vi "test.vi"() -> ()   [LabVIEW 2013]
uses:
  RydbergExpControl/red_mot_controls.ctl
  <vilib>/NI/GXML/GXML.lvlib
panel:
  out "error out":errorcluster
  in  "XML File Path":path
  in  "Inputs":T1 {"Waveform Parameters"."Degree" min=1}
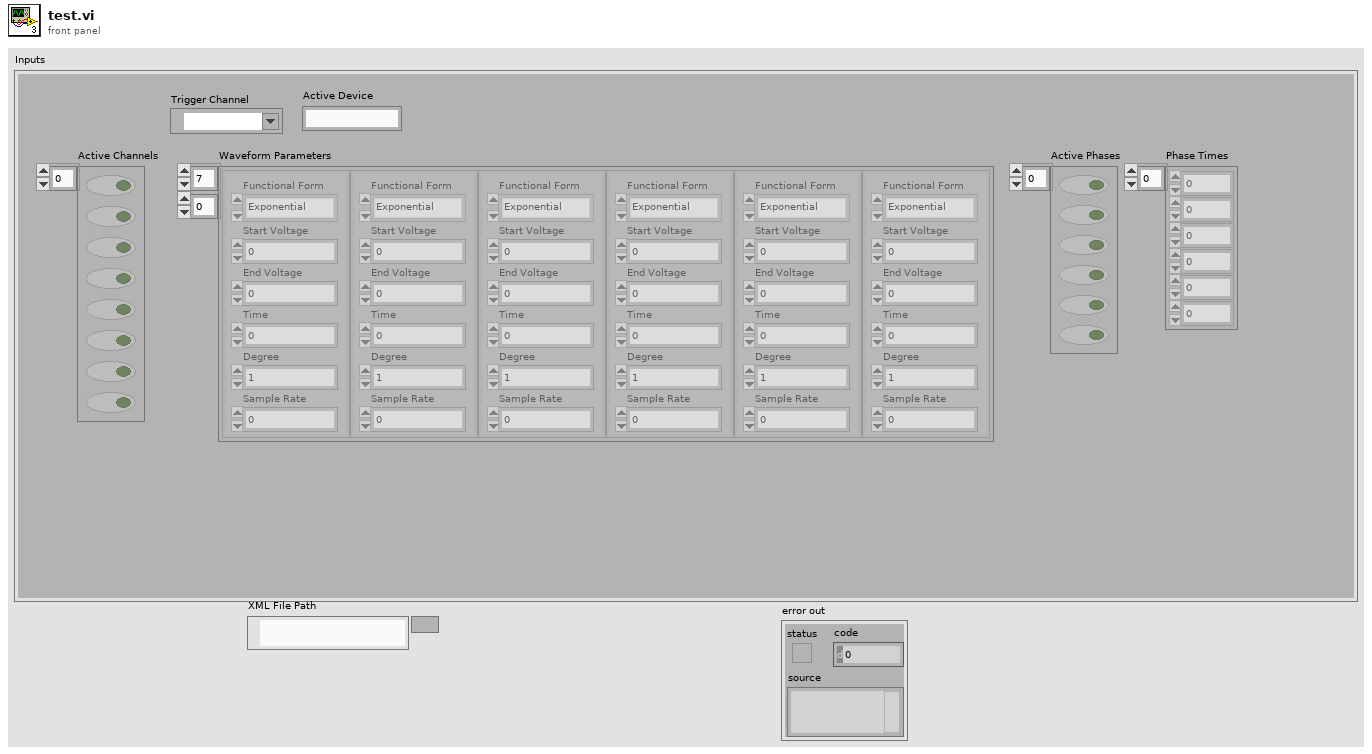
[diagram p1: front panel]
types:
  T1 = typedef "red_mot_controls.ctl" = cluster{"Active Device":string, "Active Channels":bool[], "Waveform Parameters":cluster{"Functional Form":enum16{"Polynomial", "Exponential"}, "Start Voltage":dbl, "End Voltage":dbl, "Time":dbl, "Degree":i8, "Sample Rate":dbl}[][], "Active Phases":bool[], "Phase Times":dbl[], "Trigger Channel":tag}
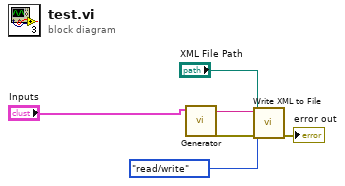
[diagram p0: block diagram]
diagram:
  n1 = call <vilib>:"Generator.vi"("Variant"="Inputs") -> ("error out"=w5:errorcluster, "XML String Out"=w4:string)  [unwired: 9 in]
  n2 = call <vilib>:"Write XML to File.vi"("error in"=w5, "file access"=enum16{"read/write", "read-only", "write-only"}."read/write", "XML File Path"="XML File Path", "XML Input"=w4) -> ("error out"=→"error out":errorcluster)  [unwired: 7 in]
